vi "Write Controls to Config File.vi"(6 "Child?":bool, 7 "section":string, 8 "Error In":errorcluster, 9 "ParentName":string, 10 "Ctl Refnum":refnum<vi>, 11 "refnum":T1) -> (0 "Error Out":errorcluster, 3 "refnum out":T1)   [LabVIEW 2018]
uses:
  <vilib>/Utility/config.llb/Config Data RefNum.ctl
  Hardware Mfg/Thorlabs Translation Stages/Controls/Translation Stage Cluster.ctl
  Controls/Translation Stage Types.ctl
  <vilib>/Utility/config.llb/Write Key (String).vi
  <vilib>/Utility/config.llb/Write Key (U32).vi
  <vilib>/Utility/config.llb/Write Key (Boolean).vi
  <vilib>/Utility/config.llb/Write Key (Double).vi
  <vilib>/Utility/config.llb/NI_LVConfig.lvlib
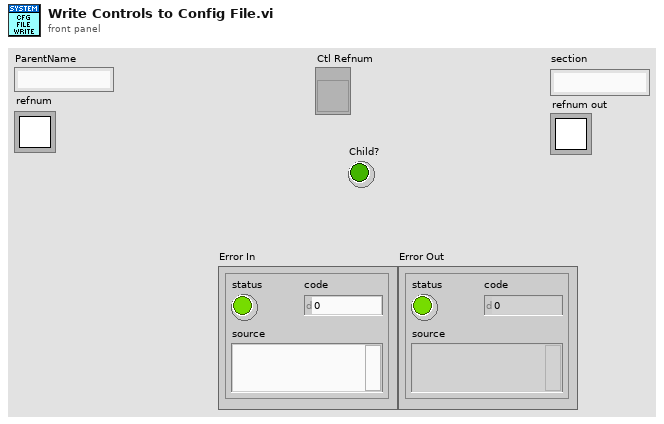
[diagram p1: front panel]
types:
  T1 = typedef "NI_LVConfig.lvlib/Config Data RefNum.ctl" = refnum<k1>
  T2 = typedef "Translation Stage Cluster.ctl" = cluster{"Position":dbl, "Is.Enabled?":bool, "Is.Connected?":bool, "Device SN":string, "AccelerationMaximum":dbl, "VelocityMaximum":dbl, "Acceleration":dbl, "Velocity":dbl, "waitTimeout (ms)":i32, "Model":T3, "Is.Homed?":bool}
  T3 = typedef "Translation Stage Types.ctl" = enum16{"None", "Thorlabs LTS", "Thorlabs MLJ"}
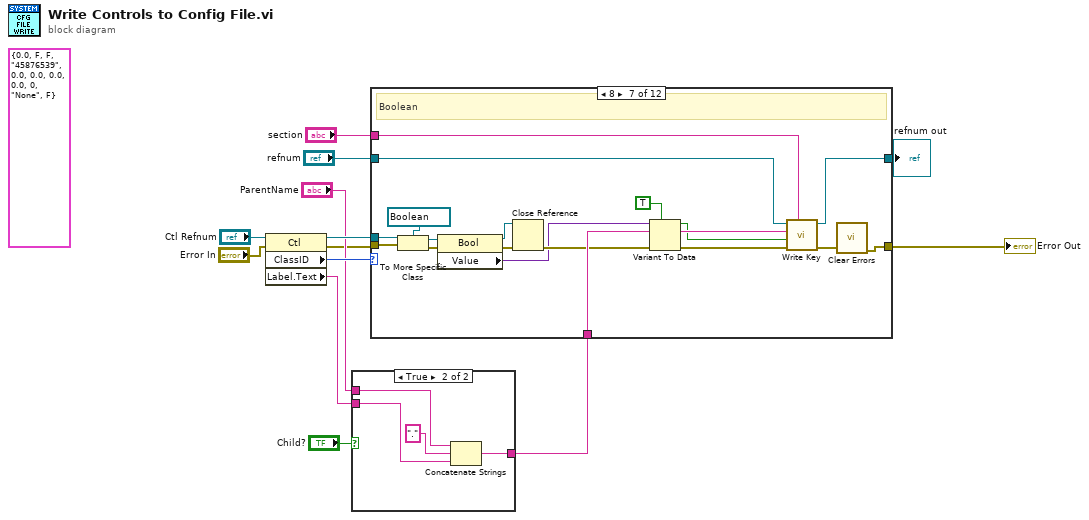
[diagram p0: block diagram]
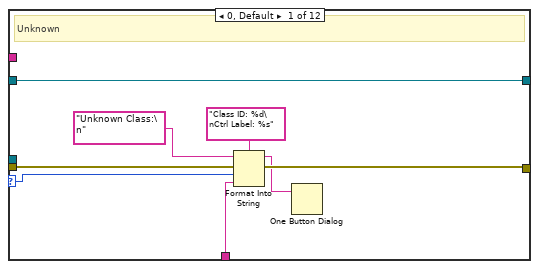
[diagram p3: hidden frame]
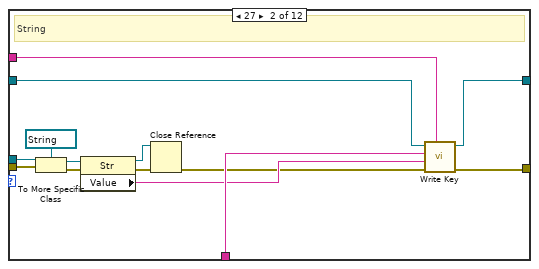
[diagram p4: hidden frame]
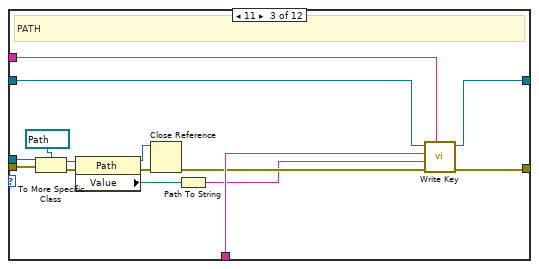
[diagram p5: hidden frame]
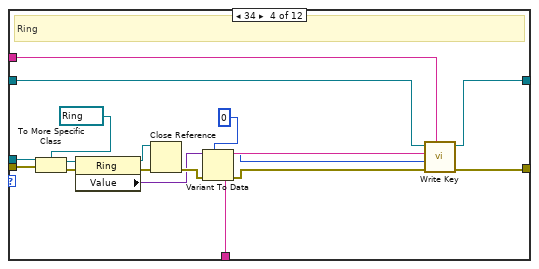
[diagram p6: hidden frame]
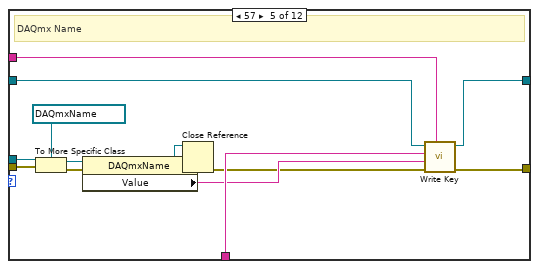
[diagram p7: hidden frame]
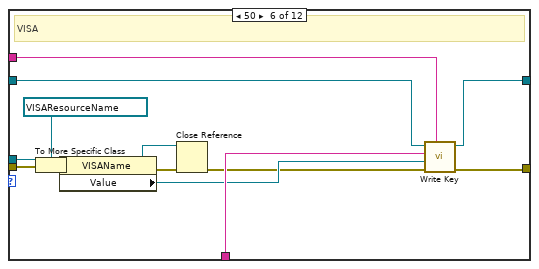
[diagram p8: hidden frame]
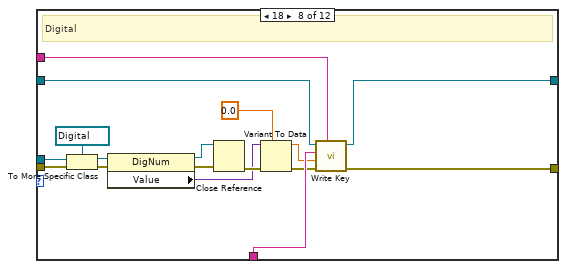
[diagram p9: hidden frame]
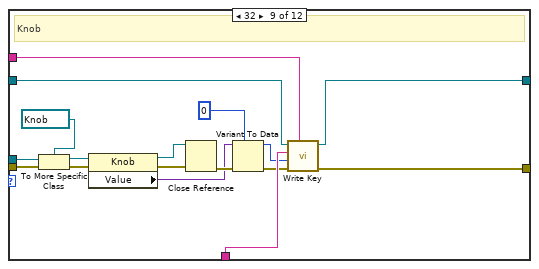
[diagram p10: hidden frame]
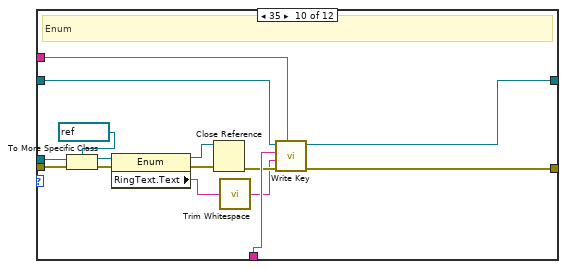
[diagram p11: hidden frame]
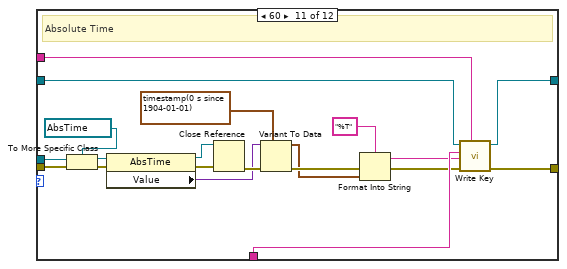
[diagram p12: hidden frame]
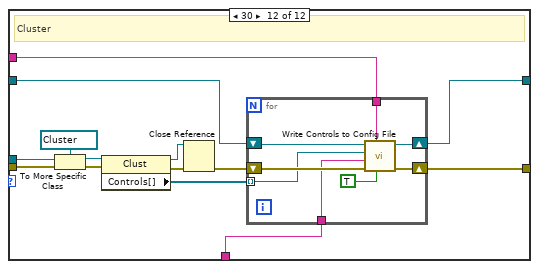
[diagram p13: hidden frame]
diagram:
  (unwired) T2 {"Position"=0.0, "Is.Enabled?"=FALSE, "Is.Connected?"=FALSE, "Device SN"="45876539", "AccelerationMaximum"=0.0, "VelocityMaximum"=0.0, "Acceleration"=0.0, "Velocity"=0.0, "waitTimeout (ms)"=0, "Model"=enum."None", "Is.Homed?"=FALSE} ("Control Param In")
  n1 = property class="Ctl"(reference="Ctl Refnum", error in="Error In") -> (reference out=w12:refnum<vi>, error out=w6:errorcluster, "ClassID"=w11:u32, "Label.Text"=w8:string)
  n2 = case shown="True" "Child?" {
    tunnel: "ParentName" -> [_ w18]
    tunnel: w8 -> [w14 w16]
    tunnel: [w14 w15] -> w3
    frame False {
    }
    frame True {
      n3 = Concatenate Strings(w18, ".", w16) -> (w15:string)
    }
  }
  n4 = case shown="8" w11 {
    selector: w11 -> [w23 _ _ _ _ _ _ _ _ _ _ _]
    tunnel: w6 -> [w21 w39 w54 w72 w86 w100 w117 w135 w152 w167 w187 w201]
    tunnel: w12 -> [_ w38 w53 w71 w85 w99 w116 w134 w151 w166 w186 w199]
    tunnel: [w20 w37 w52 w70 w84 w98 w101 w123 w141 w157 w176 w195] -> w1
    tunnel: "section" -> [_ w36 w51 w69 w83 w97 w115 w126 w144 w160 w179 w192]
    tunnel: "refnum" -> [w26 w35 w50 w68 w82 w96 w114 w125 w143 w159 w178 w194]
    tunnel: [w26 w34 w49 w67 w81 w95 w113 w124 w142 w158 w177 w193] -> w2
    tunnel: w3 -> [w22 w32 w47 w65 w79 w93 w111 w127 w145 w161 w180 w191]
    frame 0, Default {
      # "Unknown"
      n5 = Format Into String(format string="Class ID: %d\nCtrl Label: %s", initial string="Unknown Class:\n" ("string"), error in=w21, w23, w22) -> (resulting string=w19:string, error out=w20:errorcluster)
      n6 = One Button Dialog(message=w19) -> ()  [unwired: 1 in, 1 out]
    }
    frame 27 {
      # "String"
      n7 = To More Specific Class(target class=refnum<vi> refnum ("AccelerationMaximum 2"), reference=w38, error in=w39) -> (specific class reference=w30:refnum<vi>, error out=w33:errorcluster)
      n8 = property class="Str"(reference=w30, error in=w33) -> (reference out=w27:refnum<vi>, error out=w31:errorcluster, "Value"=w29:string)
      n9 = Close Reference(reference=w27, error in (no error)=w31) -> (error out=w28:errorcluster)
      n10 = call-poly <vilib>:"Write Key.vi"("section"=w36, "error in (no error)"=w28, "value"=w29, "key"=w32, "refnum"=w35) -> ("error out"=w37:errorcluster, "refnum out"=w34:T1)  [unwired: 4 in, 1 out]
    }
    frame 11 {
      # "PATH"
      n11 = To More Specific Class(target class=refnum<vi> refnum ("AccelerationMaximum 2"), reference=w53, error in=w54) -> (specific class reference=w45:refnum<vi>, error out=w48:errorcluster)
      n12 = property class="Path"(reference=w45, error in=w48) -> (reference out=w42:refnum<vi>, error out=w46:errorcluster, "Value"=w44:path)
      n13 = Close Reference(reference=w42, error in (no error)=w46) -> (error out=w43:errorcluster)
      n14 = Path To String(path=w44) -> (string=w41:string)
      n15 = call-poly <vilib>:"Write Key.vi"("section"=w51, "error in (no error)"=w43, "value"=w41, "key"=w47, "refnum"=w50) -> ("error out"=w52:errorcluster, "refnum out"=w49:T1)  [unwired: 4 in, 1 out]
    }
    frame 34 {
      # "Ring"
      n16 = To More Specific Class(target class=refnum<vi> refnum ("Trigger Operation"), reference=w71, error in=w72) -> (specific class reference=w63:refnum<vi>, error out=w66:errorcluster)
      n17 = property class="Ring"(reference=w63, error in=w66) -> (reference out=w62:refnum<vi>, error out=w64:errorcluster, "Value"=w58:variant)
      n18 = Close Reference(reference=w62, error in (no error)=w64) -> (error out=w60:errorcluster)
      n19 = Variant To Data(error in=w60, type=u32 0, Variant=w58) -> (data=w56:u32, error out=w59:errorcluster)
      n20 = call-poly <vilib>:"Write Key.vi"("section"=w69, "error in (no error)"=w59, "value"=w56, "key"=w65, "refnum"=w68) -> ("error out"=w70:errorcluster, "refnum out"=w67:T1)  [unwired: 4 in, 1 out]
    }
    frame 57 {
      # "DAQmx Name"
      n21 = To More Specific Class(target class=refnum<vi> refnum ("Analog Out Channel"), reference=w85, error in=w86) -> (specific class reference=w77:refnum<vi>, error out=w80:errorcluster)
      n22 = property class="DAQmxName"(reference=w77, error in=w80) -> (reference out=w74:refnum<vi>, error out=w78:errorcluster, "Value"=w76:string)
      n23 = Close Reference(reference=w74, error in (no error)=w78) -> (error out=w75:errorcluster)
      n24 = call-poly <vilib>:"Write Key.vi"("section"=w83, "error in (no error)"=w75, "value"=w76, "key"=w79, "refnum"=w82) -> ("error out"=w84:errorcluster, "refnum out"=w81:T1)  [unwired: 4 in, 1 out]
    }
    frame 50 {
      # "VISA"
      n25 = To More Specific Class(target class=refnum<vi> refnum ("Controller VISA Ref"), reference=w99, error in=w100) -> (specific class reference=w91:refnum<vi>, error out=w94:errorcluster)
      n26 = property class="VISAName"(reference=w91, error in=w94) -> (reference out=w88:refnum<vi>, error out=w92:errorcluster, "Value"=w90:refnum<visa-resource-name>)
      n27 = Close Reference(reference=w88, error in (no error)=w92) -> (error out=w89:errorcluster)
      n28 = call-poly <vilib>:"Write Key.vi"("section"=w97, "error in (no error)"=w89, "value"=w90, "key"=w93, "refnum"=w96) -> ("error out"=w98:errorcluster, "refnum out"=w95:T1)  [unwired: 4 in, 1 out]
    }
    frame 8 {
      # "Boolean"
      n29 = To More Specific Class(target class=refnum<vi> refnum ("AccelerationMaximum 2"), reference=w116, error in=w117) -> (specific class reference=w109:refnum<vi>, error out=w112:errorcluster)
      n30 = property class="Bool"(reference=w109, error in=w112) -> (reference out=w107:refnum<vi>, error out=w110:errorcluster, "Value"=w105:variant)
      n31 = Close Reference(reference=w107, error in (no error)=w110) -> (error out=w108:errorcluster)
      n32 = Variant To Data(error in=w108, type=TRUE, Variant=w105) -> (data=w103:bool, error out=w106:errorcluster)
      n33 = call-poly <vilib>:"Write Key.vi"("section"=w115, "error in (no error)"=w106, "value"=w103, "key"=w111, "refnum"=w114) -> ("error out"=w102:errorcluster, "refnum out"=w113:T1)  [unwired: 4 in, 1 out]
      n34 = call <vilib>:"Clear Errors.vi"("error in (no error)"=w102) -> ("error out"=w101:errorcluster)  [unwired: 5 in, 1 out]
    }
    frame 18 {
      # "Digital"
      n35 = To More Specific Class(target class=refnum<vi> refnum ("AccelerationMaximum 2"), reference=w134, error in=w135) -> (specific class reference=w131:refnum<vi>, error out=w132:errorcluster)
      n36 = property class="DigNum"(reference=w131, error in=w132) -> (reference out=w129:refnum<vi>, error out=w130:errorcluster, "Value"=w121:variant)
      n37 = Close Reference(reference=w129, error in (no error)=w130) -> (error out=w128:errorcluster)
      n38 = Variant To Data(error in=w128, type=0.0, Variant=w121) -> (data=w119:dbl, error out=w122:errorcluster)
      n39 = call-poly <vilib>:"Write Key.vi"("section"=w126, "error in (no error)"=w122, "value"=w119, "key"=w127, "refnum"=w125) -> ("error out"=w123:errorcluster, "refnum out"=w124:T1)  [unwired: 4 in, 1 out]
    }
    frame 32 {
      # "Knob"
      n40 = To More Specific Class(target class=refnum<vi> refnum ("Zoom Factor"), reference=w151, error in=w152) -> (specific class reference=w149:refnum<vi>, error out=w150:errorcluster)
      n41 = property class="Knob"(reference=w149, error in=w150) -> (reference out=w147:refnum<vi>, error out=w148:errorcluster, "Value"=w139:variant)
      n42 = Close Reference(reference=w147, error in (no error)=w148) -> (error out=w146:errorcluster)
      n43 = Variant To Data(error in=w146, type=u32 0, Variant=w139) -> (data=w137:u32, error out=w140:errorcluster)
      n44 = call-poly <vilib>:"Write Key.vi"("section"=w144, "error in (no error)"=w140, "value"=w137, "key"=w145, "refnum"=w143) -> ("error out"=w141:errorcluster, "refnum out"=w142:T1)  [unwired: 4 in, 1 out]
    }
    frame 35 {
      # "Enum"
      n45 = To More Specific Class(target class=refnum<vi> refnum ("Enum"), reference=w166, error in=w167) -> (specific class reference=w164:refnum<vi>, error out=w165:errorcluster)
      n46 = property class="Enum"(reference=w164, error in=w165) -> (reference out=w162:refnum<vi>, error out=w163:errorcluster, "RingText.Text"=w154:string)
      n47 = Close Reference(reference=w162, error in (no error)=w163) -> (error out=w155:errorcluster)
      n48 = call <vilib>:"Trim Whitespace.vi"("string"=w154) -> ("trimmed string"=w153:string)  [unwired: 1 in]
      n49 = call-poly <vilib>:"Write Key.vi"("section"=w160, "error in (no error)"=w155, "value"=w153, "key"=w161, "refnum"=w159) -> ("error out"=w157:errorcluster, "refnum out"=w158:T1)  [unwired: 4 in, 1 out]
    }
    frame 60 {
      # "Absolute Time"
      n50 = To More Specific Class(target class=refnum<vi> refnum ("AccelerationMaximum 2"), reference=w186, error in=w187) -> (specific class reference=w184:refnum<vi>, error out=w185:errorcluster)
      n51 = property class="AbsTime"(reference=w184, error in=w185) -> (reference out=w182:refnum<vi>, error out=w183:errorcluster, "Value"=w174:variant)
      n52 = Close Reference(reference=w182, error in (no error)=w183) -> (error out=w181:errorcluster)
      n53 = Variant To Data(error in=w181, type=timestamp(0 s since 1904-01-01), Variant=w174) -> (data=w168:timestamp, error out=w175:errorcluster)
      n54 = Format Into String(format string="%T", error in=w175, w168) -> (resulting string=w172:string, error out=w173:errorcluster)  [unwired: 1 in]
      n55 = call-poly <vilib>:"Write Key.vi"("section"=w179, "error in (no error)"=w173, "value"=w172, "key"=w180, "refnum"=w178) -> ("error out"=w176:errorcluster, "refnum out"=w177:T1)  [unwired: 4 in, 1 out]
    }
    frame 30 {
      # "Cluster"
      n56 = To More Specific Class(target class=refnum<vi> refnum ("Cluster Ref In"), reference=w199, error in=w201) -> (specific class reference=w197:refnum<vi>, error out=w198:errorcluster)
      n57 = property class="Clust"(reference=w197, error in=w198) -> (reference out=w189:refnum<vi>, error out=w196:errorcluster, "Controls[]"=w188:refnum<vi>[])
      n58 = Close Reference(reference=w189, error in (no error)=w196) -> (error out=w190:errorcluster)
      n59 = for {
        tunnel: w192 -> [w205]
        tunnel: w191 -> [w204]
        shift-right: [w208] -> w195
        shift-left: w190 -> [w209]
        shift-right: [w206] -> w193
        shift-left: w194 -> [w207]
        tunnel: w188 -> [w202] mode=indexing
        n60 = call "Write Controls to Config File.vi"("Child?"=TRUE, "section"=w205, "Error In"=w209, "ParentName"=w204, "Ctl Refnum"=w202, "refnum"=w207) -> ("Error Out"=w208:errorcluster, "refnum out"=w206:T1)  [unwired: 4 in]
      }
    }
  }
  "Error Out" <- w1
  "refnum out" <- w2
